vi "data_entry_numeric.vi"(7 "caller":refnum<vi>, 8 "error in (no error)":errorcluster, 11 "configuration":T2) -> (0 "error out":errorcluster, 2 "data_entry out":dbl, 3 "dialog_selection":T1=enum."button_2")   [LabVIEW 2015, in "lv-dialog-interfaces.lvlib"]
uses:
  lv-dialog-interfaces.lvlib
  <userlib>/antonio-alexander/lv-dialog/api/v1/public/_controls/selection.ctl
  private/_controls/dialog_type.ctl
  private/_controls/hmi_references.ctl
  private/_controls/configuration.ctl
  <vilib>/event_ctls.llb/eventvkey.ctl
  <userlib>/antonio-alexander/lv-dialog/api/v1/v1.lvlib
panel:
  out "dialog":string
  in  "data_entry":dbl
  in  "button 1":bool
  in  "button_2":bool
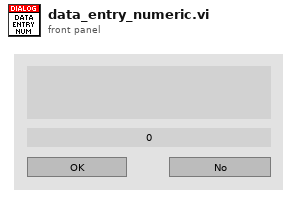
[diagram p1: front panel]
types:
  T1 = typedef "lv-dialog.lvlib/v1.lvlib/selection.ctl" = enum16{"null", "panel_closed", "button_1", "button_2", "button_3", "cancelled"}
  T2 = cluster{"dialog_text":string, "boolean_text_1":string, "boolean_text_2":string}
  T3 = typedef "lv-dialog-interfaces.lvlib/dialog_type.ctl" = enum16{"null", "one_button", "two_button", "three_button", "confirmation", "busy_wait", "error", "busy_wait_embed", "combo_box", "data_entry_string", "data_entry_numeric"}
  T4 = typedef "lv-dialog-interfaces.lvlib/configuration.ctl" = cluster{"dialog_text":string, "boolean_text_1":string, "boolean_text_2":string, "boolean_text_3":string, "inner_color":u32, "outer_color":u32, "wait_s":dbl, "error_status":bool, "error_source":string, "error_details":string, "string []":string[], "custom_entry":bool, "confirmation_text":string}
  T5 = typedef "lv-dialog-interfaces.lvlib/hmi_references.ctl" = cluster{"vi_reference":refnum<vi>, "caller":refnum<vi>, "dialog":refnum<vi>, "button_1":refnum<vi>, "button_2":refnum<vi>, "button_3":refnum<vi>, "busy":refnum<vi>, "error_glyph":refnum<vi>, "error_source":refnum<vi>, "error_text":refnum<vi>, "combo_box":refnum<vi>}
  T6 = typedef "eventvkey.ctl" = enum16{"ASCII", "Enter", "Return", "Shift", "Ctrl", "Alt", "Cmd", "Opt", "Caps", "NumLock", "Clear", "Break", "Up", "Down", "Left", "Right", "Insert", "Delete", "Home", "End", "PageUp", "PageDown", "Escape", "Help", "Pause", "ScrollLock", "F1", "F2", "F3", "F4", "F5", "F6", "F7", "F8", "F9", "F10", "F11", "F12", "F13", "F14", "F15", "F16", "F17", "F18", "F19", "F20", "F21", "F22", "F23", "F24", "Play", "VolumeUp", "VolumeDown", "Mute", "Two Byte Char"}
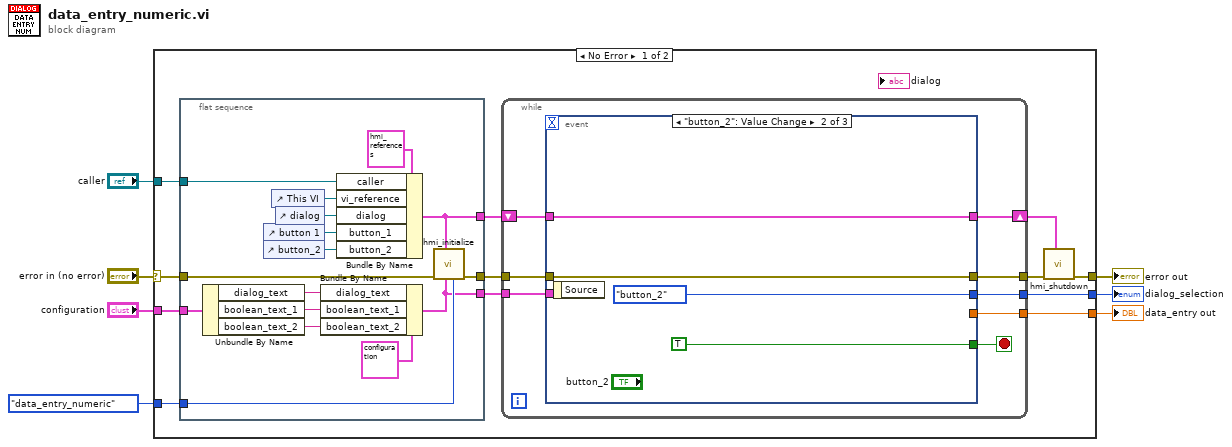
[diagram p0: block diagram]
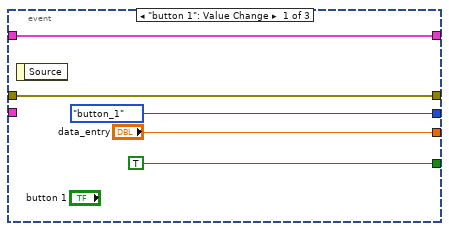
[diagram p2: hidden frame]
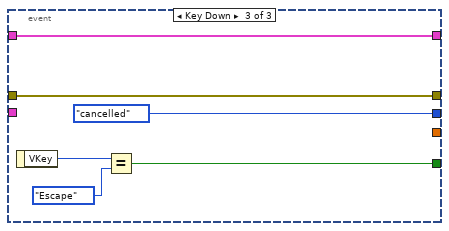
[diagram p3: hidden frame]
diagram:
  n1 = case shown="No Error" "error in (no error)" {
    selector: "error in (no error)" -> [w17 w59]
    tunnel: [w18 w59] -> w7
    tunnel: [w16 _] -> w1
    tunnel: "caller" -> [w15 _]
    tunnel: "configuration" -> [w8 _]
    tunnel: dialog_type."data_entry_numeric" ("dialog_type") -> [w14 _]
    tunnel: [w9 _] -> w3
    frame No Error {
      n2 = flat-sequence {
        tunnel: w17 -> [w28]
        tunnel: [w29] -> w13
        tunnel: [w23] -> w12
        tunnel: w15 -> [w33]
        tunnel: w14 -> [w27]
        tunnel: [w26] -> w11
        tunnel: w8 -> [w25]
        frame #0 {
          n3 = Unbundle By Name(w25) -> ("dialog_text"=w22:string, "boolean_text_1"=w21:string, "boolean_text_2"=w20:string)
          n4 = control-ref of="button 1"() -> (w32:refnum<vi>)
          n5 = control-ref of="button_2"() -> (w31:refnum<vi>)
          n6 = control-ref of="This VI"() -> (w34:refnum<vi>)
          n7 = control-ref of="dialog"() -> (w30:refnum<vi>)
          n8 = Bundle By Name(cluster=T4 {"dialog_text"="", "boolean_text_1"="", "boolean_text_2"="", "boolean_text_3"="", "inner_color"=16711680, "outer_color"=6618880, "wait_s"=nan, "error_status"=FALSE, "error_source"="", "error_details"="", "string []"=[], "custom_entry"=FALSE, "confirmation_text"=""} ("configuration"), "dialog_text"=w22, "boolean_text_1"=w21, "boolean_text_2"=w20) -> (w23:T4)
          n9 = Bundle By Name(cluster=T5 {"vi_reference"=refnum, "caller"=refnum, "dialog"=refnum, "button_1"=refnum, "button_2"=refnum, "button_3"=refnum, "busy"=refnum, "error_glyph"=refnum, "error_source"=refnum, "error_text"=refnum, "combo_box"=refnum} ("references"), "caller"=w33, "vi_reference"=w34, "dialog"=w30, "button_1"=w32, "button_2"=w31) -> (w26:T5)
          n10 = call "hmi_initialize.vi"("dialog_type"=w27, "configuration"=w23, "references"=w26, "error in (no error)"=w28) -> ("error out"=w29:errorcluster)  [unwired: 7 in]
        }
      }
      n11 = while {
        tunnel: w13 -> [w40]
        tunnel: [w43] -> w16
        tunnel: w12 -> [w41]
        tunnel: [w39] -> w19
        shift-right: [w37] -> w10
        shift-left: w11 -> [w38]
        tunnel: [w36] -> w9
        stop <- w42 stop-if-true
        n12 = event shown="[1] \"button_2\": Value Change" {
          selector: _ -> [_ _ _]
          dyn-events: _ -> [_ _ _]
          timeout: _ -> [_ _ _]
          tunnel: [selection."button_1" ("dialog_selection") selection."button_2" ("dialog_selection") selection."cancelled" ("dialog_selection")] -> w43
          tunnel: [TRUE TRUE w55] -> w42
          tunnel: w41 -> [_ _ _]
          tunnel: w40 -> [w47 w50 w57]
          tunnel: [w47 w50 w57] -> w39
          tunnel: w38 -> [w45 w49 w56]
          tunnel: [w45 w49 w56] -> w37
          tunnel: ["data_entry" _ _] -> w36
          event "button 1": Value Change {
            n13 = event-data() -> ()  [unwired: 1 in, 1 out]
          }
          event "button_2": Value Change {
            n14 = event-data() -> ()  [unwired: 1 in, 1 out]
          }
          event Key Down {
            n15 = event-data() -> ("VKey"=w54:T6)  [unwired: 1 in]
            n16 = Equal?(x=w54, y=eventvkey."Escape" ("VKey")) -> (x = y?=w55:bool)
          }
        }
      }
      n17 = call "hmi_shutdown.vi"("references"=w10, "error in (no error)"=w19) -> ("error out"=w18:errorcluster)  [unwired: 9 in]
    }
    frame Error {
    }
  }
  "error out" <- w7
  "data_entry out" <- w3
  "dialog_selection" <- w1
